vi "PH_Beckhoff_10BB_Plus.declare digital InputTags.vi"(2 "Digital Inputs to be inverted [#s separated by ::]":string, 3 "Instance Name":string="<Instance Name>") -> (0 "Digital Inputs":T2, 1 "Description":string)   [LabVIEW 2014, in "PH_Beckhoff_10BB_Plus.lvlib"]
uses:
  PH_Beckhoff_10BB_Plus.lvlib
  PH_Beckhoff/PH_Beckhoff.Digital Inputs.ctl
  PH_Beckhoff/PH_Beckhoff.lvlib
  PH_Beckhoff_Common/PH_Beckhoff_Common.lvlib
panel:
  in  "Digital Input Value":T1
  out "Right Size?":bool
  # "Let this VI run to check the size!"
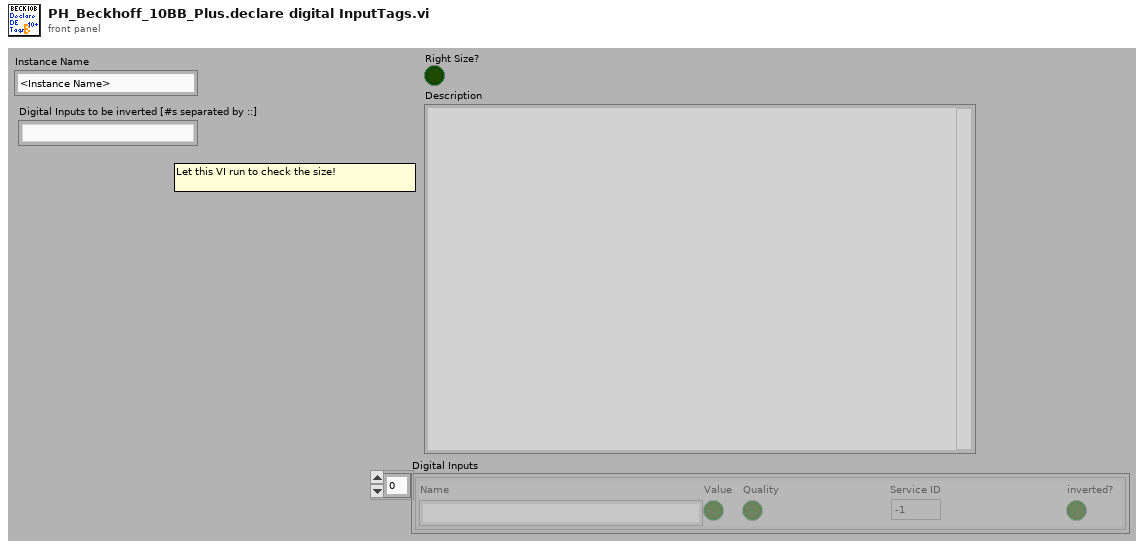
[diagram p1: front panel]
types:
  T1 = cluster{"Name":string, "Value":bool, "Quality":bool, "Service ID":i32, "inverted?":bool}
  T2 = typedef "PH_Beckhoff.lvlib/PH_Beckhoff.Digital Inputs.ctl" = cluster{"Name":string, "Value":bool, "Quality":bool, "Service ID":i32, "inverted?":bool}[]
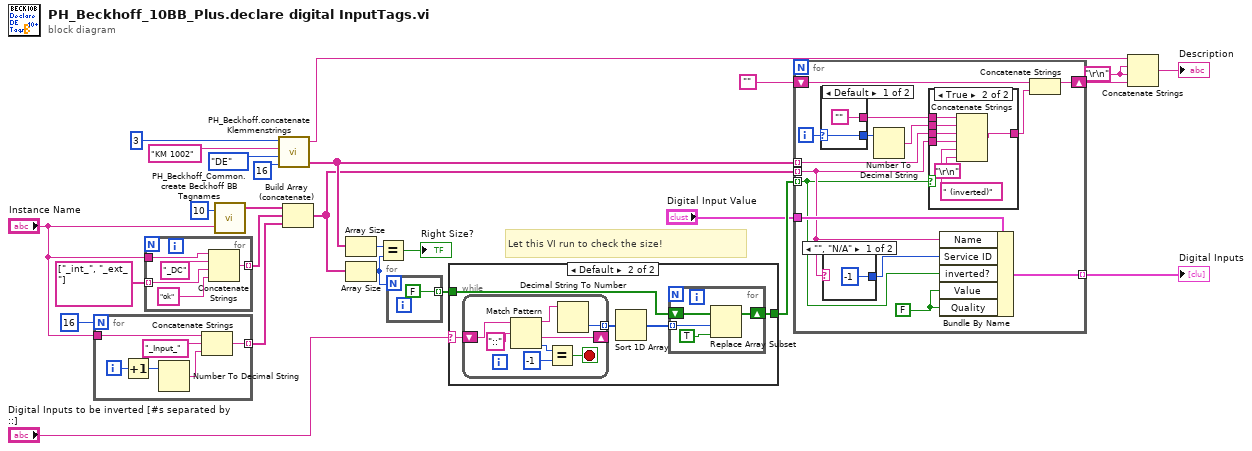
[diagram p0: block diagram]
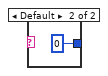
[diagram p3: hidden frame]
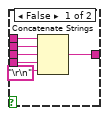
[diagram p4: hidden frame]
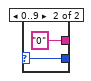
[diagram p5: hidden frame]
diagram:
  w18 = "\r\n"
  # "Let this VI run to check the size!"
  n1 = for {
    N: 16 -> [_]
    tunnel: "Instance Name" -> [w32]
    tunnel: [w31] -> w26 mode=indexing
    i -> [w28]
    n2 = Increment(x=w28) -> (x+1=w29:i32)
    n3 = Number To Decimal String(number=w29) -> (decimal integer string=w27:string)  [unwired: 1 in]
    n4 = Concatenate Strings(w32, "_Input_" ("string"), w27) -> (w31:string)
  }
  n5 = for {
    tunnel: "Instance Name" -> [w37]
    tunnel: string[] ["_int_", "_ext_"] -> [w34] mode=indexing
    tunnel: [w36] -> w25 mode=indexing
    n6 = Concatenate Strings(w37, "_DC" ("string"), w34, "ok" ("string")) -> (w36:string)
  }
  n7 = call "PH_Beckhoff_Common.create Beckhoff BB Tagnames.vi"("#"=10, "Instance Name"="Instance Name") -> ("Input Tags"=w6:string[])  [unwired: 2 out]
  n8 = call "PH_Beckhoff.concatenate Klemmenstrings.vi"("# of In- or Outputs"=16, "Type"=enum16{"AE", "AA", "DE", "DA"}."DE", "Klemmenname"="KM 1002", "Quantity"=3 ("size(s)")) -> ("concatenated string array"=w13:string[], "\"<Type>: <Quantity> x <Klemmenname>\""=w15:string)  [unwired: 1 out]
  n9 = Build Array (concatenate)(w6, w25, w26) -> (w3:string[])
  n10 = Array Size(array=w13) -> (size(s)=w12:i32)
  n11 = Array Size(array=w3) -> (size(s)=w5:i32)
  n12 = Equal?(x=w12, y=w5) -> (x = y?=→"Right Size?":bool)
  n13 = for {
    N: w5 -> [_]
    tunnel: [FALSE] -> w10 mode=indexing
  }
  n14 = case shown="Default" "Digital Inputs to be inverted [#s separated by ::]" {
    selector: "Digital Inputs to be inverted [#s separated by ::]" -> [_ w44]
    tunnel: w10 -> [w39 w41]
    tunnel: [w39 w40] -> w4
    frame "", "N/A" {
    }
    frame Default {
      n15 = while {
        shift-right: [w51] -> _
        shift-left: w44 -> [w56]
        tunnel: [w49] -> w43 mode=indexing
        stop <- w52 stop-if-true
        n16 = Match Pattern(string=w56, regular expression="::") -> (before substring=w50:string, after substring=w51:string, offset past match=w54:i32)  [unwired: 1 in, 1 out]
        n17 = Equal?(x=w54, y=-1) -> (x = y?=w52:bool)
        n18 = Decimal String To Number(string=w50) -> (number=w49:i32)  [unwired: 2 in, 1 out]
      }
      n19 = Sort 1D Array(array=w43) -> (sorted array=w42:i32[])
      n20 = for {
        tunnel: w42 -> [w46] mode=indexing
        shift-right: [w47] -> w40
        shift-left: w41 -> [w48]
        n21 = Replace Array Subset(array=w48, new element=TRUE ("new element/subarray"), index=w46) -> (w47:bool[])
      }
    }
  }
  n22 = for {
    tunnel: w3 -> [w61] mode=indexing
    tunnel: w13 -> [w66] mode=indexing
    shift-right: [w64] -> w19
    shift-left: "" -> [w63]
    tunnel: w4 -> [w59] mode=indexing
    tunnel: "Digital Input Value" -> [w62]
    tunnel: [w57] -> w1 mode=indexing
    i -> [w70]
    w58 = FALSE ("Quality")
    n23 = case shown="Default" w70 {
      selector: w70 -> [w86 w89]
      tunnel: [w86 w89] -> w69
      tunnel: ["" "0"] -> w68
      frame Default {
      }
      frame 0..9 {
      }
    }
    n24 = case shown="\"\", \"N/A\"" w61 {
      tunnel: [-1 0] -> w60
      frame "", "N/A" {
      }
      frame Default {
      }
    }
    n25 = Number To Decimal String(number=w69) -> (decimal integer string=w67:string)  [unwired: 1 in]
    n26 = case shown="True" w59 {
      tunnel: w68 -> [w78 w85]
      tunnel: w67 -> [w77 w84]
      tunnel: w66 -> [w76 w83]
      tunnel: w61 -> [w75 w82]
      tunnel: [w73 w80] -> w65
      frame False {
        n27 = Concatenate Strings(w78, w77, w76, w75, "\r\n") -> (w73:string)
      }
      frame True {
        n28 = Concatenate Strings(w85, w84, w83, w82, " (inverted)", "\r\n") -> (w80:string)
      }
    }
    n29 = Bundle By Name(cluster=w62, "Name"=w61, "Service ID"=w60, "inverted?"=w59, "Value"=w58, "Quality"=w58) -> (w57:T1)
    n30 = Concatenate Strings(w63, w65) -> (w64:string)
  }
  "Digital Inputs" <- w1
  n31 = Concatenate Strings(w15, w18, w18, w19) -> (→"Description":string)
